vi "ch act update.vi"(7 "cmd":T2=enum."initial", 8 "error in (no error)":errorcluster, 10 "현재채널번호":u8, 11 "Cluster":T1) -> (0 "error out":errorcluster)   [LabVIEW 2019]
uses:
  cmd_ch act.ctl
  def_chact.ctl
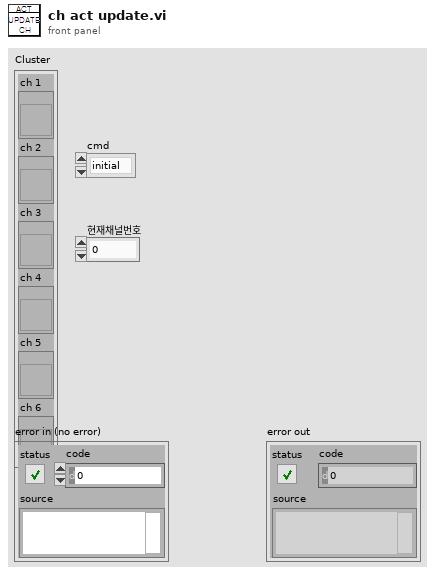
[diagram p1: front panel]
types:
  T1 = typedef "def_chact.ctl" = cluster{"ch 1":refnum<vi>, "ch 2":refnum<vi>, "ch 3":refnum<vi>, "ch 4":refnum<vi>, "ch 5":refnum<vi>, "ch 6":refnum<vi>}
  T2 = typedef "cmd_ch act.ctl" = enum16{"open", "initial", "update"}
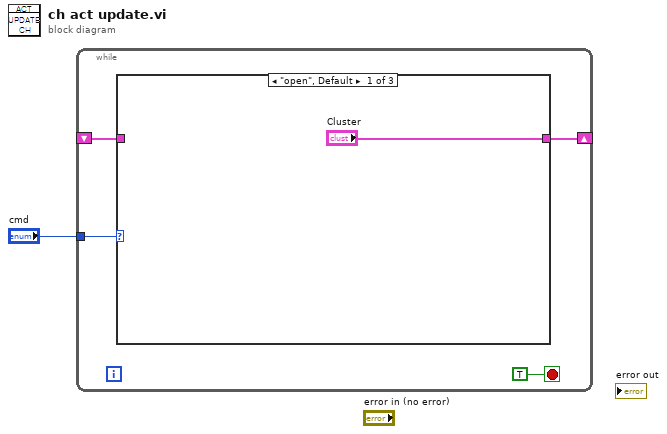
[diagram p0: block diagram]
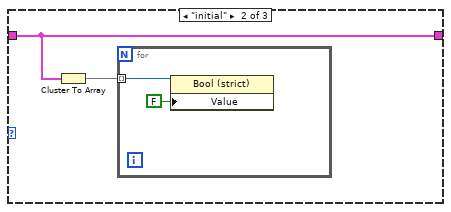
[diagram p2: hidden frame]
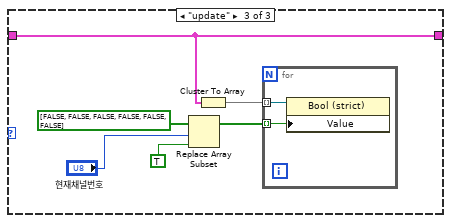
[diagram p3: hidden frame]
diagram:
  n1 = while {
    tunnel: "cmd" -> [w4]
    shift-right: [w3] -> _
    shift-left: _ -> [w2]
    stop <- TRUE stop-if-true
    n2 = case shown="\"open\", Default" w4 {
      tunnel: ["Cluster" w8 w13] -> w3
      tunnel: w2 -> [_ w8 w13]
      frame "open", Default {
      }
      frame "initial" {
        n3 = Cluster To Array(cluster=w8) -> (array=w7:refnum<vi>[])
        n4 = for {
          tunnel: w7 -> [w10] mode=indexing
          n5 = property class="Bool (strict)"(reference=w10, "Value"=FALSE) -> ()  [unwired: 1 in, 2 out]
        }
      }
      frame "update" {
        n6 = Replace Array Subset(array=bool[] [FALSE, FALSE, FALSE, FALSE, FALSE, FALSE], new element=TRUE, index="현재채널번호") -> (w11:bool[])
        n7 = Cluster To Array(cluster=w13) -> (array=w12:refnum<vi>[])
        n8 = for {
          tunnel: w12 -> [w18] mode=indexing
          tunnel: w11 -> [w17] mode=indexing
          n9 = property class="Bool (strict)"(reference=w18, "Value"=w17) -> ()  [unwired: 1 in, 2 out]
        }
      }
    }
  }
